vi "Write Scaled Data.vi"(7 "Component Index":i32, 8 "error in (no error)":errorcluster, 9 "Scaled Data":dbl[](array[numeric]), 10 "Parameters":string[](array[string]), 11 "1553 Board in":refnum<class "1553 Session.lvclass">) -> (0 "error out":errorcluster, 3 "1553 Board out":refnum<class "1553 Session.lvclass">)   [LabVIEW 2020, in "BCI-1553 API.lvlib" / "1553 Session.lvclass"]
doc: "Writes data that is in engineering units down to a component in a 1553 Session. The engineering data is rescaled to raw values based on the parameter scaling information. The component index determines which component will be targeted for the new parameter value."
uses:
  1553 Session.lvclass
  1553 Session.lvclass/1553 Session.ctl
  1553 Component/1553 Component.lvclass
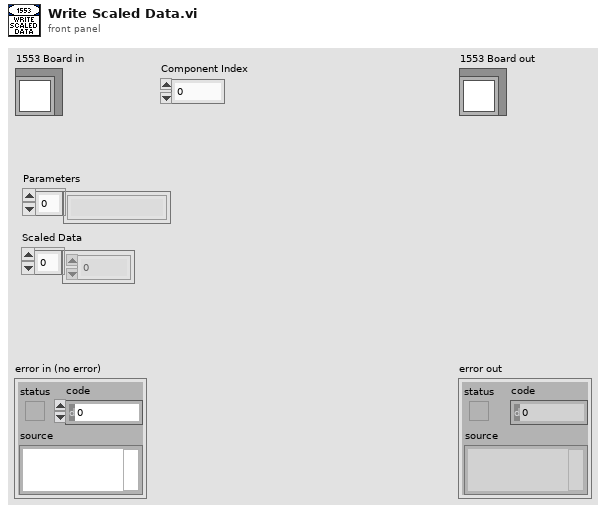
[diagram p1: front panel]
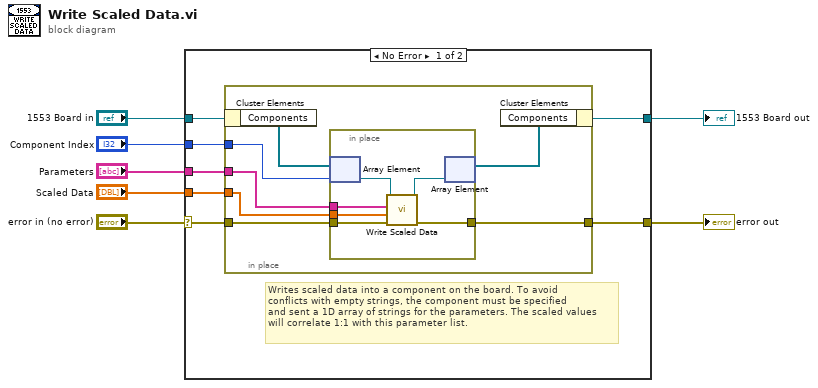
[diagram p0: block diagram]
diagram:
  n1 = case shown="No Error" "error in (no error)" {
    selector: "error in (no error)" -> [w14 w29]
    tunnel: [w13 w29] -> w5
    tunnel: [w11 w28] -> w6
    tunnel: "1553 Board in" -> [w12 w28]
    tunnel: "Component Index" -> [w10 _]
    tunnel: "Parameters" -> [w9 _]
    tunnel: "Scaled Data" -> [w8 _]
    frame No Error {
      # "Writes scaled data into a component on the board. To avoid\nconflicts with empty strings, the component must be specified\nand sent a 1D array of strings for the parameters. The scaled values\nwill correlate 1:1 with this parameter list."
      n2 = in-place {
        in-place-border: w14 -> [w21]
        in-place-border: [w20] -> w13
        in-place-border: w10 -> [w17]
        in-place-border: w9 -> [w16]
        in-place-border: w8 -> [w15]
        n3 = in-place-cluster #1(w12) -> ("Components"=w19:refnum<class "1553 Component.lvclass">[])
        n4 = in-place {
          in-place-border: w21 -> [w25]
          in-place-border: [w24] -> w20
          in-place-border: w16 -> [w22]
          in-place-border: w15 -> [w23]
          n5 = in-place-array #2(w19, w17) -> (w27:refnum<class "1553 Component.lvclass">)
          n6 = call-dynamic "Write Scaled Data.vi"("error in (no error)"=w25, "Scaled Data"=w23, "Parameters"=w22, "1553 Component in"=w27) -> ("error out"=w24:errorcluster, "1553 Component out"=w26:refnum<class "1553 Component.lvclass">)  [unwired: 6 in]
          n7 = in-place-array #2(w26) -> (w18:refnum<class "1553 Component.lvclass">[])  [unwired: 1 out]
        }
        n8 = in-place-cluster #1("Components"=w18) -> (w11:refnum<class "1553 Session.lvclass">)
      }
    }
    frame Error {
    }
  }
  "error out" <- w5
  "1553 Board out" <- w6
